vi "Label 2 Dataset Transaction Id.vi"(10 "Label":string) -> (2 "Dataset Trans Id":T1)   [LabVIEW 2009]
uses:
  Dataset Transaction Id.ctl
  Dataset Source.ctl
  Dataset Type.ctl
  Apps/Yes No Button.ctl
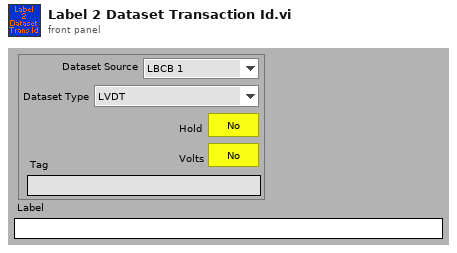
[diagram p1: front panel]
types:
  T1 = typedef "Dataset Transaction Id.ctl" = cluster{"Dataset Source":T2, "Dataset Type":T3, "Hold":T4, "Volts":T4, "Tag":string}
  T2 = typedef "Dataset Source.ctl" = enum16{"LBCB 1", "LBCB 2", "Combined", "External Sensors"}
  T3 = typedef "Dataset Type.ctl" = enum16{"LVDT", "Load Cell", "Actuator Command", "Servo Error", "Displacement Command", "Displacement", "Force"}
  T4 = typedef "Yes No Button.ctl" = bool
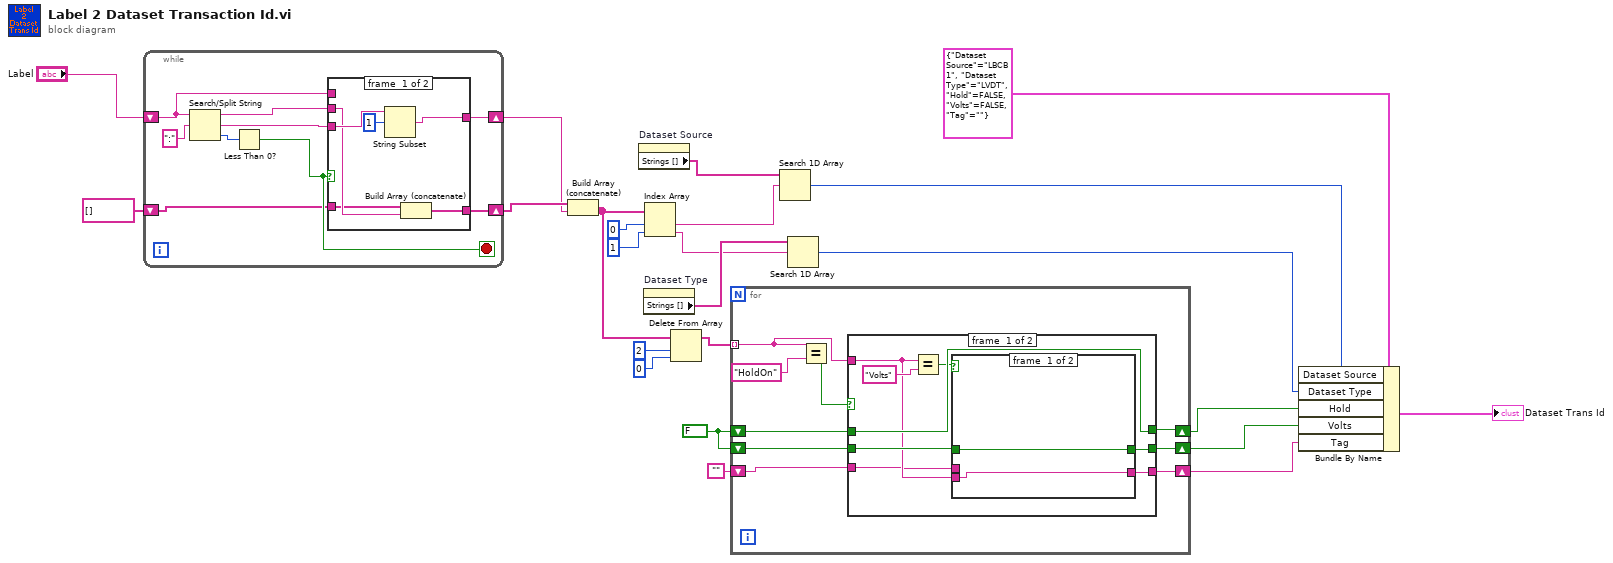
[diagram p0: block diagram]
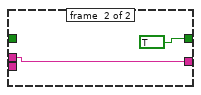
[diagram p2: hidden frame]
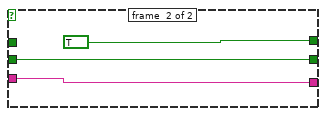
[diagram p3: hidden frame]
diagram:
  w9 = FALSE
  n1 = while {
    shift-right: [w30] -> w1
    shift-left: "Label" -> [w27]
    shift-right: [w26] -> w2
    shift-left: string[] [] -> [w25]
    stop <- w28 stop-if-true
    n2 = Search/Split String(string=w27, search string/char (-)=":") -> (substring before match=w29:string, match + rest of string=w31:string, offset of match=w32:i32)  [unwired: 1 in]
    n3 = Less Than 0?(x=w32) -> (x < 0?=w28:bool)
    n4 = case shown="True" w28 {
      tunnel: w31 -> [w38 _]
      tunnel: [w36 w40] -> w30
      tunnel: w29 -> [w35 _]
      tunnel: w27 -> [_ w40]
      tunnel: [w34 w39] -> w26
      tunnel: w25 -> [w33 w39]
      frame #0 {
        n5 = String Subset(string=w38, offset (0)=1) -> (substring=w36:string)  [unwired: 1 in]
        n6 = Build Array (concatenate)(w33, w35) -> (w34:string[])
      }
      frame #1 {
      }
    }
  }
  n7 = Build Array (concatenate)(w2, w1) -> (w3:string[])
  n8 = property on="Dataset Source" class="Enum (strict)"() -> ("Strings []"=w18:string[])  [unwired: 2 in, 2 out]
  n9 = property on="Dataset Type" class="Enum (strict)"() -> ("Strings []"=w15:string[])  [unwired: 2 in, 2 out]
  n10 = Index Array(array=w3, index #1=0 ("index"), index #2=1 ("index")) -> (element #1=w17:string, element #2=w14:string)
  n11 = Delete From Array(array=w3, length=2, index=0) -> (array with subset deleted=w10:string[])  [unwired: 1 out]
  n12 = for {
    tunnel: w10 -> [w49] mode=indexing
    shift-right: [w48] -> w7
    shift-left: w9 -> [w47]
    shift-right: [w46] -> w6
    shift-left: w9 -> [w45]
    shift-right: [w44] -> w5
    shift-left: "" -> [w43]
    n13 = Equal?(x=w49, y="HoldOn") -> (x = y?=w41:bool)
    n14 = case shown="True" w41 {
      tunnel: [w57 TRUE] -> w48
      tunnel: w47 -> [w57 _]
      tunnel: w49 -> [w52 _]
      tunnel: [w54 w63] -> w46
      tunnel: w45 -> [w53 w63]
      tunnel: [w51 w62] -> w44
      tunnel: w43 -> [w50 w62]
      frame #0 {
        n15 = Equal?(x=w52, y="Volts") -> (x = y?=w55:bool)
        n16 = case shown="True" w55 {
          tunnel: [w59 TRUE] -> w54
          tunnel: w53 -> [w59 _]
          tunnel: w52 -> [w58 _]
          tunnel: [w58 w60] -> w51
          tunnel: w50 -> [_ w60]
          frame #0 {
          }
          frame #1 {
          }
        }
      }
      frame #1 {
      }
    }
  }
  n17 = Search 1D Array(1D array=w18, element=w17) -> (index of element=w16:i32)  [unwired: 1 in]
  n18 = Search 1D Array(1D array=w15, element=w14) -> (index of element=w13:i32)  [unwired: 1 in]
  n19 = Bundle By Name(cluster=T1 {"Dataset Source"=enum."LBCB 1", "Dataset Type"=enum."LVDT", "Hold"=FALSE, "Volts"=FALSE, "Tag"=""} ("Dataset Trans Id"), "Dataset Source"=w16, "Dataset Type"=w13, "Hold"=w7, "Volts"=w6, "Tag"=w5) -> (→"Dataset Trans Id":T1)
